vi "COMSelect_86.vi"(7 "error in (no error)":errorcluster) -> (0 "error out":errorcluster, 2 "return count":u32=1, 3 "COM Port Selected":string="USB0::0x2457::0x1022::NI-VISA-20002::RAW")   [LabVIEW 2026]
doc: "COMSelect.vi detects all instruments with an ASRL instrument name on all local and remote machines, and allows manual selection of a particular serial port. The output of this function can then be passed into a VISA Open function to generate a VISA Reference"
panel:
  in  "USB port":u16(ring)
  in  "OK Button":bool
  # "Select COM Port and Press OK"
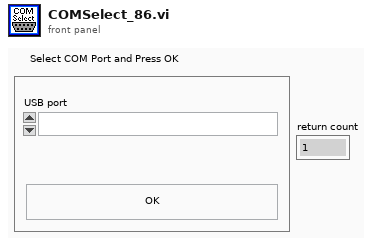
[diagram p1: front panel]
types:
  T1 = enum16{"Detect Instruments", "Open Front Panel", "Wait for User Input", "Close"}
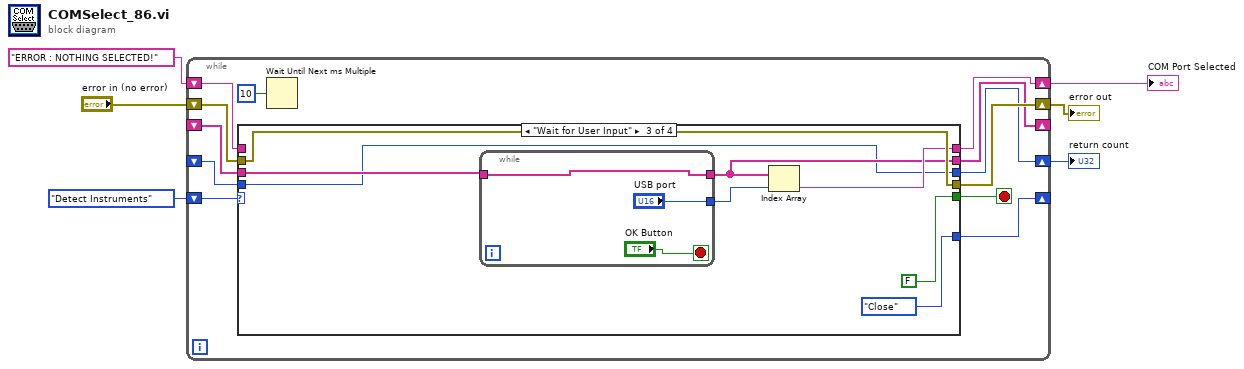
[diagram p0: block diagram]
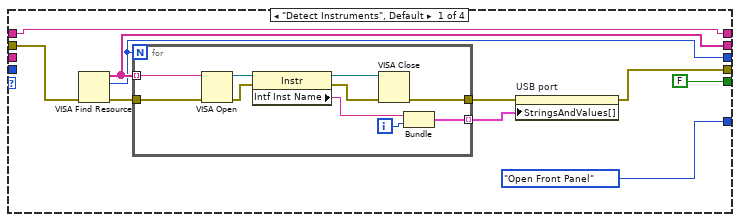
[diagram p2: hidden frame]
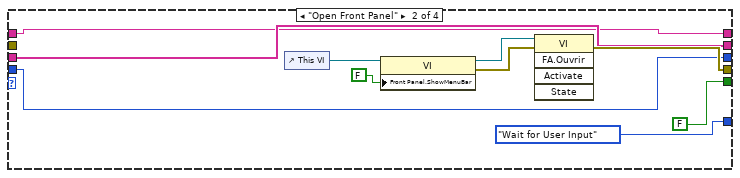
[diagram p3: hidden frame]
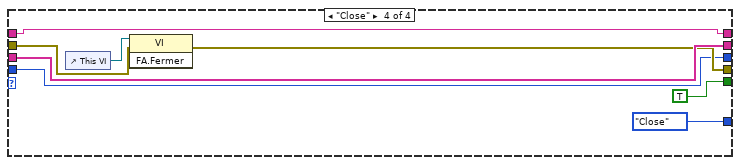
[diagram p4: hidden frame]
diagram:
  n1 = while {
    shift-right: [w17] -> _
    shift-left: T1."Detect Instruments" -> [w18]
    shift-right: [w15] -> w4
    shift-left: "error in (no error)" -> [w16]
    shift-right: [w13] -> _
    shift-left: _ -> [w12]
    shift-right: [w10] -> w3
    shift-left: "ERROR : NOTHING SELECTED!" -> [w9]
    shift-right: [w8] -> w1
    shift-left: _ -> [w7]
    stop <- w11 stop-if-true
    n2 = case shown="\"Wait for User Input\"" w18 {
      tunnel: [T1."Open Front Panel" T1."Wait for User Input" T1."Close" T1."Close"] -> w17
      tunnel: w16 -> [w25 _ w53 w62]
      tunnel: [w23 w48 w53 w61] -> w15
      tunnel: [w22 w45 w50 w65] -> w13
      tunnel: w12 -> [_ w45 w51 w65]
      tunnel: [FALSE FALSE FALSE TRUE] -> w11
      tunnel: [w20 w44 w52 w64] -> w10
      tunnel: w9 -> [w20 w44 _ w64]
      tunnel: [w19 w39 w49 w60] -> w8
      tunnel: w7 -> [_ w39 w49 w60]
      frame "Detect Instruments", Default {
        n3 = VISA Find Resource(8:w25) -> (0:w27:errorcluster, 2:w19:u32, 3:w22:string[])  [unwired: 1 in, 1 out]
        n4 = for {
          N: w19 -> [_]
          tunnel: w22 -> [w38] mode=indexing
          tunnel: w27 -> [w36]
          tunnel: [w30] -> w28 mode=indexing
          tunnel: [w29] -> w24
          i -> [w32]
          n5 = VISA Open(error in (no error)=w36, VISA resource name=w38) -> (VISA resource name=w37:refnum<visa-resource-name>, error out=w35:errorcluster)  [unwired: 3 out]
          n6 = property class="Instr"(reference=w37, error in=w35) -> (reference out=w33:refnum<visa-resource-name>, error out=w34:errorcluster, "Intf Inst Name"=w31:string)
          n7 = VISA Close(VISA resource name=w33, error in (no error)=w34) -> (error out=w29:errorcluster)
          n8 = Bundle("Intf Inst Name"=w31, w32) -> (w30:cluster{"Intf Inst Name":string, i32})  [unwired: 1 out]
        }
        n9 = property on="USB port" class="MDér (strict)"(error in=w24, "StringsAndValues[]"=w28) -> (error out=w23:errorcluster)  [unwired: 1 in, 1 out]
      }
      frame "Open Front Panel" {
        n10 = control-ref of="This VI"() -> (w41:refnum<vi>)
        n11 = property class="VI"(reference=w41, "Front Panel.ShowMenuBar"=FALSE ("Front Panel Window:Show Menu Bar")) -> (reference out=w42:refnum<vi>, error out=w43:errorcluster)  [unwired: 1 in]
        n12 = invoke class="VI" method="FA.Ouvrir"(reference=w42, error in=w43) -> (error out=w48:errorcluster)  [unwired: 3 in, 4 out]
      }
      frame "Wait for User Input" {
        n13 = while {
          tunnel: ["USB port"] -> w56
          tunnel: [w58] -> w50
          tunnel: w51 -> [w58]
          stop <- "OK Button" stop-if-true
        }
        n14 = Index Array(array=w50, index=w56) -> (element=w52:string)
      }
      frame "Close" {
        n15 = control-ref of="This VI"() -> (w63:refnum<vi>)
        n16 = invoke class="VI" method="FA.Fermer"(reference=w63, error in=w62) -> (error out=w61:errorcluster)  [unwired: 1 in, 2 out]
      }
    }
    n17 = Wait Until Next ms Multiple(millisecond multiple=u32 10) -> ()  [unwired: 1 out]
  }
  "error out" <- w4
  "COM Port Selected" <- w3
  "return count" <- w1
